vi "Complex Voltage(V) to Mean Power (dBm).vi"(11 "Y":cdb[](array[numeric])) -> (1 "Numeric":dbl)   [LabVIEW 2014]
uses:
  <vilib>/Analysis/baseanly.llb/Mean (DBL).vi
  <vilib>/Analysis/NI_AALBase.lvlib
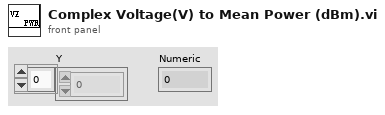
[diagram p1: front panel]
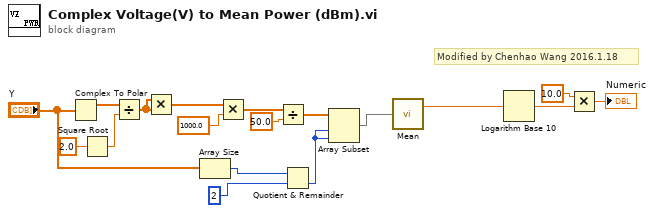
[diagram p0: block diagram]
diagram:
  # "Modified by Chenhao Wang 2016.1.18"
  n1 = Complex To Polar(r * e^(i*theta)="Y") -> (r=w16:dbl[])  [unwired: 1 out]
  n2 = Square Root(x=2.0) -> (sqrt(x)=w17:dbl)
  n3 = Divide(x=w16, y=w17) -> (x/y=w15:dbl[])
  n4 = Multiply(x=w15, y=w15) -> (x*y=w14:dbl[])
  n5 = Array Size(array="Y") -> (size(s)=w5:i32)
  n6 = Multiply(x=w14, y=1000.0) -> (x*y=w11:dbl[])
  n7 = Divide(x=w11, y=50.0) -> (x/y=w2:dbl[])
  n8 = Quotient & Remainder(x=w5, y=2) -> (floor(x/y)=w3:i32)  [unwired: 1 out]
  n9 = Array Subset(array=w2, index=w3, length=w3) -> (w1:dbl[])
  n10 = call-poly <vilib>:"Mean.vi"("X"=w1) -> ("mean"=w10:dbl)  [unwired: 1 out]
  n11 = Logarithm Base 10(1:w10) -> (0:w9:dbl)
  n12 = Multiply(x=10.0, y=w9) -> (x*y=→"Numeric":dbl)
